vi "TestExecuteValueChangeSubscription_RejectRepeats.vi"(8 "error in (no error)":errorcluster, 11 "TestCase in":refnum<class "TestSubscriptionPolicy.lvclass">) -> (0 "error out":errorcluster, 3 "TestCase out":refnum<class "TestSubscriptionPolicy.lvclass">)   [LabVIEW 2017, in "TestSubscriptionPolicy.lvclass"]
uses:
  TestSubscriptionPolicy.lvclass
  gpm_packages/@cs/mva-core/Source/IMediator/ISubscriptionPolicy/ISubscriptionPolicy.lvclass
  gpm_packages/@cs/mva-core/Source/SubscriptionPolicy/ValueChangeSubscription/ValueChangeSubscription.lvclass
  gpm_packages/@cs/transport/Source/Concrete/QueueTransport/QueueTransport.lvclass
  C:/Git/mva-framework/gpm_packages/@cs/transport/Source/ITransport/ITransport.lvclass
  C:/Git/mva-framework/Source/Framework/IMediator/ISubscriptionPolicy/ISubscriptionPolicy.lvclass
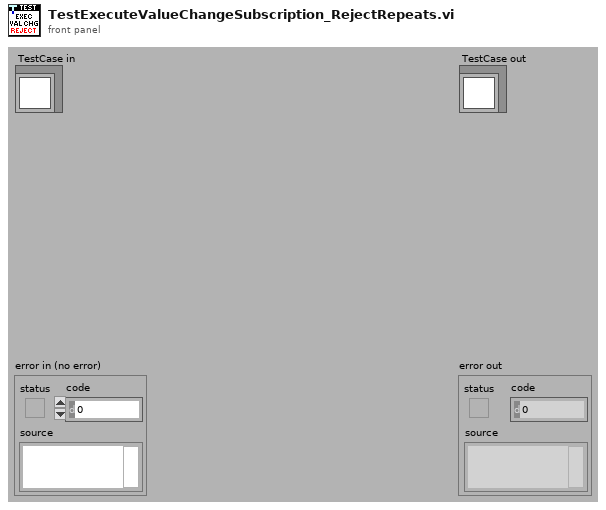
[diagram p1: front panel]
types:
  T1 = typedef "IMediator.lvlib/ISubscriptionPolicy.lvclass/ISubscriptionPolicy Reference.ctl" = refnum<data-value>
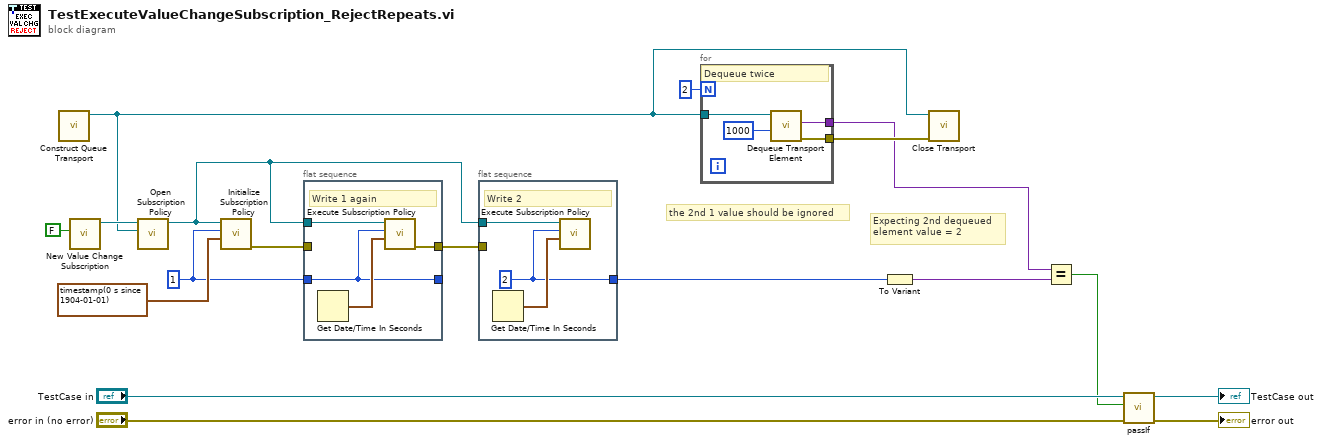
[diagram p0: block diagram]
diagram:
  w9 = 1
  # "the 2nd 1 value should be ignored"
  # "Expecting 2nd dequeued\nelement value = 2"
  n1 = call "Construct Queue Transport.vi"() -> ("QueueTransport"=w1:refnum<class "QueueTransport.lvclass">)  [unwired: 10 in, 1 out]
  n2 = call "New Value Change Subscription.vi"("Ignore Past Updates? (F)"=FALSE) -> ("ValueChangeSubscription Out"=w13:refnum<class "ValueChangeSubscription.lvclass">)  [unwired: 10 in]
  n3 = call "Open Subscription Policy.vi"("Transport"=w1, "SubscriptionPolicy"=w13) -> ("Subscription Policy"=w6:T1)  [unwired: 8 in, 1 out]
  n4 = call "Initialize Subscription Policy.vi"("Last Publish Time"=timestamp(0 s since 1904-01-01), "Last Topic Value"=w9, "Subscription Policy"=w6) -> ("Error Out (Unsubscribe?)"=w7:errorcluster)  [unwired: 7 in, 1 out]
  n5 = flat-sequence {
    tunnel: w9 -> [w20]
    tunnel: w6 -> [w21]
    tunnel: w7 -> [_]
    tunnel: [w20] -> _
    tunnel: [w19] -> w3
    frame #0 {
      # "Write 1 again"
      n6 = Get Date/Time In Seconds() -> (seconds since 1Jan1904=w22:timestamp)
      n7 = call "Execute Subscription Policy.vi"("Publish Time"=w22, "New Topic Value"=w20, "Subscription Policy"=w21) -> ("error out (Unsubscribe?)"=w19:errorcluster)  [unwired: 7 in, 1 out]
    }
  }
  n8 = flat-sequence {
    tunnel: w6 -> [w24]
    tunnel: [w23] -> w5
    tunnel: w3 -> [_]
    frame #0 {
      w23 = 2
      # "Write 2"
      n9 = Get Date/Time In Seconds() -> (seconds since 1Jan1904=w25:timestamp)
      n10 = call "Execute Subscription Policy.vi"("Publish Time"=w25, "New Topic Value"=w23, "Subscription Policy"=w24) -> ()  [unwired: 7 in, 2 out]
    }
  }
  n11 = for {
    N: 2 -> [_]
    tunnel: [w28] -> w2
    tunnel: [w27] -> w14
    tunnel: w1 -> [w26]
    # "Dequeue twice"
    n12 = call "Dequeue Transport Element.vi"("Timeout In ms (-1)"=1000, "QueueTransport"=w26) -> ("error out"=w27:errorcluster, "Data"=w28:variant)  [unwired: 6 in, 2 out]
  }
  n13 = To Variant(anything=w5) -> (Variant=w11:variant)
  n14 = call-dynamic "Close Transport.vi"("error in (no error)"=w14, "QueueTransport"=w1) -> ()  [unwired: 9 in, 1 out]
  n15 = Equal?(x=w2, y=w11) -> (x = y?=w8:bool)
  n16 = call-dynamic "passIf.vi"("error in (no error)"="error in (no error)", "pass"=w8, "TestCase in"="TestCase in") -> ("error out"=→"error out":errorcluster, "TestCase out"=→"TestCase out":refnum<class "TestSubscriptionPolicy.lvclass">)  [unwired: 7 in]
